vi "Get Connection String.vi"(4 "Error In":errorcluster, 7 "Config Data_DB_ADO_Jet in":refnum<class "Config Data_DB_ADO_Jet.lvclass">) -> (0 "Error Out":errorcluster, 2 "Connection String":string, 3 "Config Data_DB_ADO_Jet out":refnum<class "Config Data_DB_ADO_Jet.lvclass">)   [LabVIEW 2014, in "Config Data.lvlib" / "Config Data_DB_ADO_Jet.lvclass"]
uses:
  Config Data_DB_ADO_Jet.lvclass
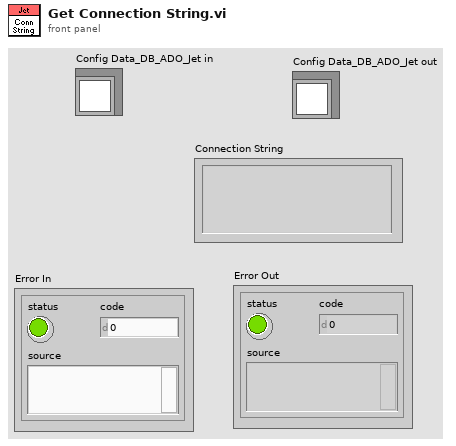
[diagram p1: front panel]
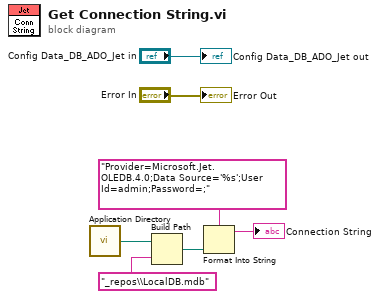
[diagram p0: block diagram]
diagram:
  n1 = call <vilib>:"Application Directory.vi"() -> ("Application Directory"=w2:path)
  n2 = Build Path(base path=w2, name or relative path="_repos\\LocalDB.mdb") -> (appended path=w4:path)
  n3 = Format Into String(format string="Provider=Microsoft.Jet.OLEDB.4.0;Data Source='%s';User Id=admin;Password=;", w4) -> (resulting string=→"Connection String":string)  [unwired: 2 in, 1 out]
  "Error Out" <- "Error In"
  "Config Data_DB_ADO_Jet out" <- "Config Data_DB_ADO_Jet in"
